vi "MockbusTest.vi"() -> ()   [LabVIEW 2016]
uses:
  Common_RT_ILC/DataTypes/ILCTelemetry.ctl
  Common_RT_ILC/DataTypes/ILCScanRates.ctl
  Common_RT_HPILC/DataTypes/HPTelemetry.ctl
  Common_RT_Modbus/DataTypes/RxFrame.ctl
  Common_RT_HealthAndStatus/RTHealthAndStatus/RTHealthAndStatus.lvclass
  MyHealthAndStatusReadFIFO/MyHealthAndStatusReadFIFO.lvclass
  D:/Code/Common_RT_FPGA/IReadU32FIFO/IReadU32FIFO.lvclass
  MyHealthAndStatusWriteFIFO/MyHealthAndStatusWriteFIFO.lvclass
  D:/Code/Common_RT_FPGA/IWriteU64FIFO/IWriteU64FIFO.lvclass
  ModbusFactory/ModbusFactory.lvclass
  D:/Code/Common_RT_Modbus/IModbusFactory/IModbusFactory.lvclass
  SubnetFactory/SubnetFactory.lvclass
  Subnet/DataTypes/SubnetSettings.ctl
  Common_RT_HPILC/DataTypes/HPSettings.ctl
  Common_RT_ILC/DataTypes/ILCSettings.ctl
  Common_RT_Modbus/IModbusFactory/IModbusFactory.lvclass
  Common_RT_MTILC/DataTypes/MTSettings.ctl
  Common_RT_MDILC/DataTypes/MDSettings.ctl
  Common_RT_MIILC/DataTypes/MISettings.ctl
  ModbusFactory/ModbusFactory.lvclass/ModbusFactory.ctl
  MyHealthAndStatusWriteFIFO/MyHealthAndStatusWriteFIFO.lvclass/MyHealthAndStatusWriteFIFO.ctl
  MyHealthAndStatusReadFIFO/MyHealthAndStatusReadFIFO.lvclass/MyHealthAndStatusReadFIFO.ctl
  Common_RT_HealthAndStatus/RTHealthAndStatus/RTHealthAndStatus.lvclass/RTHealthAndStatus.ctl
  Subnet/Subnet.lvclass/Subnet.ctl
  Common_RT_ILC/ILC/ILC.lvclass/ILC.ctl
  Common_RT_Modbus/DynamicFrameParser/DynamicFrameParser.lvclass
  Common_RT_HPILC/HPILC/HPILC.lvclass/HPILC.ctl
  Common_RT_HPILC/HPILC/HPILC.lvclass
  D:/Code/Common_RT_ILC/ILC/ILC.lvclass
  <vilib>/FPGAPlugInAG/cRIO-9038/niLvFpga_Open_cRIO-9038.vi
  <vilib>/rvi/interface/common/dynamic/niFpgaDynamicAddResources.vi
  <vilib>/FPGAPlugInAG/Dynamic/niLvFpga_Abort_Dynamic.vi
  <vilib>/FPGAPlugInAG/Dynamic/niLvFpga_Reset_Dynamic.vi
  <vilib>/FPGAPlugInAG/Dynamic/niLvFpga_Run_Dynamic.vi
  <vilib>/Utility/error.llb/Error Cluster From Error Code.vi
  <vilib>/rvi/errors/niLvFpgaAdjustHostInterfaceError.vi
  <vilib>/FPGAPlugInAG/Dynamic/niLvFpga_Close_Dynamic.vi
  <vilib>/rvi/interface/nirviOpenFPGA/nirviOpenFPGA.xnode
  FPGA Bitfiles/mockbusTesting.lvbitx
  FPGA/mockbusTesting.vi
  <vilib>/rvi/interface/nirviMethod/nirviMethod.xnode
  <vilib>/rvi/interface/nirviCloseFPGA/nirviCloseFPGA.xnode
  Subnet/Subnet.lvclass
  Common_RT_Modbus/IModbus/IModbus.lvclass
  Common_RT_ILC/RTILC.lvlib
  Common_RT_HPILC/RTHPILC.lvlib
  <vilib>/rvi/errors/niLvFpgaMergeErrorWithErrorCode.vi
  <vilib>/FPGAPlugInAG/Dynamic/niLvFpga_ReadFifo_Dynamic.vi
  Common_RT_MIILC/RTMIILC.lvlib
  Common_RT_MDILC/RTMDILC.lvlib
  Common_RT_MTILC/RTMTILC.lvlib
  <vilib>/FPGAPlugInAG/Dynamic/niLvFpga_WriteFifo_Dynamic.vi
  Common_RT_ILC/ILC/ILC.lvclass
  Common_RT_Modbus/RTModbus.lvlib
panel:
  out "CRCIssues":T1[](array[typedef]) {"Data" format="%02x"}
  in  "BroadcastCounter":u8
  in  "Command.Steps":i8
  out "Telemetry":T2
  out "InvalidCRC":i32
  out "ValidCRC":i32
  out "Array":T3[](array[typedef]) {"ADCScanRate" items=["50 Hz"=0, "60 Hz"=1, "100 Hz"=2, "120 Hz"=3, "200 Hz"=4, "240 Hz"=5, "300 Hz"=6, "400 Hz"=7, "480 Hz"=8, "600 Hz"=9, "1200 Hz"=10, "2400 Hz"=11, "4800 Hz"=12, "No Change"=255]}
  out "Port 2 Status Bits":u64 format="%016b"
  out "Port 2 Frames Received":i64
  out "Port 2 Bytes Received":i64
  out "Port 2 Frames Transmitted":i64
  out "Port 2 Bytes Transmitted":i64
  in  "Boolean":bool
  out "Port 1 Status Bits":u64 format="%016b"
  out "error out":errorcluster
  out "Port 1 Frames Received":i64
  out "Port 1 Bytes Received":i64
  out "Port 1 Frames Transmitted":i64
  out "Port 1 Bytes Transmitted":i64
  # "Port 1 = Modbus"
  # "Port 2 = Mockbus"
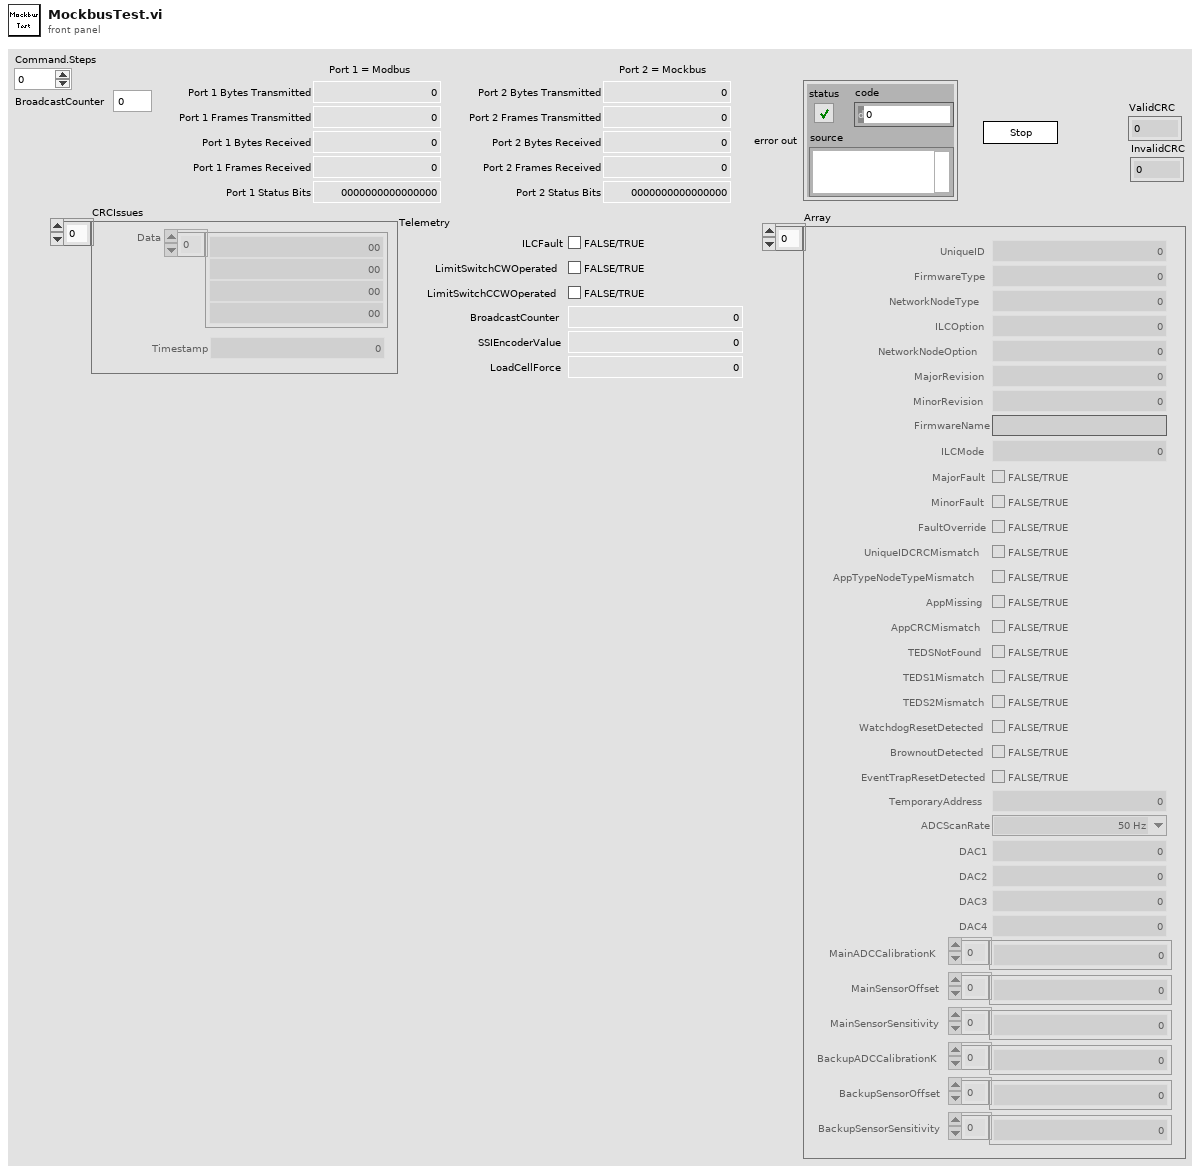
[diagram p1: front panel]
types:
  T1 = typedef "RTModbus.lvlib/RxFrame.ctl" = cluster{"Data":u8[], "Timestamp":u64}
  T2 = typedef "RTHPILC.lvlib/HPTelemetry.ctl" = cluster{"ILCFault":bool, "LimitSwitchCWOperated":bool, "LimitSwitchCCWOperated":bool, "BroadcastCounter":u8, "SSIEncoderValue":i32, "LoadCellForce":sgl}
  T3 = typedef "RTILC.lvlib/ILCTelemetry.ctl" = cluster{"UniqueID":u64, "FirmwareType":u8, "NetworkNodeType":u8, "ILCOption":u8, "NetworkNodeOption":u8, "MajorRevision":u8, "MinorRevision":u8, "FirmwareName":string, "ILCMode":u16, "MajorFault":bool, "MinorFault":bool, "FaultOverride":bool, "UniqueIDCRCMismatch":bool, "AppTypeNodeTypeMismatch":bool, "AppMissing":bool, "AppCRCMismatch":bool, "TEDSNotFound":bool, "TEDS1Mismatch":bool, "TEDS2Mismatch":bool, "WatchdogResetDetected":bool, "BrownoutDetected":bool, "EventTrapResetDetected":bool, "TemporaryAddress":u8, "ADCScanRate":T4, "DAC1":u16, "DAC2":u16, "DAC3":u16, "DAC4":u16, "MainADCCalibrationK":sgl[], "MainSensorOffset":sgl[], "MainSensorSensitivity":sgl[], "BackupADCCalibrationK":sgl[], "BackupSensorOffset":sgl[], "BackupSensorSensitivity":sgl[]}
  T4 = typedef "RTILC.lvlib/ILCScanRates.ctl" = u8
  T5 = typedef "RTHPILC.lvlib/HPSettings.ctl" = cluster{"ILCSettings":T6, "ID":i16, "ReferencePosition":i32}
  T6 = typedef "RTILC.lvlib/ILCSettings.ctl" = cluster{"Subnet":u8, "Address":u8}
  T7 = typedef "SubnetSettings.ctl" = cluster{"HPs":T5[], "ModbusFactory":refnum<class "IModbusFactory.lvclass">, "Port":i32, "MTs":T8[], "MDs":T9[], "MIs":T10[]}
  T8 = typedef "RTMTILC.lvlib/MTSettings.ctl" = cluster{"ILCSettings":T6, "ID":i16}
  T9 = typedef "RTMDILC.lvlib/MDSettings.ctl" = cluster{"ILCSettings":T6, "ID":i16}
  T10 = typedef "RTMIILC.lvlib/MISettings.ctl" = cluster{"ILCSettings":T6, "ID":i16}
  T11 = typedef "SubnetData.ctl" = cluster{"SubnetConstants":T12, "SubnetCommand":T15, "SubnetTelemetry":T16}
  T12 = typedef "SubnetConstants.ctl" = cluster{"Modbus":refnum<class "IModbus.lvclass">, "HPs":refnum<class "HPILC.lvclass">[], "AddressToActuator":T13[], "MTs":refnum<class "MTILC.lvclass">[], "MDs":refnum<class "MDILC.lvclass">[], "MIs":refnum<class "MIILC.lvclass">[]}
  T13 = typedef "ILCIndexData.ctl" = cluster{"ILCTypes":T14, "Index":i32}
  T14 = typedef "ILCTypes.ctl" = enum16{"Undefined", "SAA", "DAA", "HP", "MT", "MD", "MI"}
  T15 = typedef "SubnetCommand.ctl" = cluster{"BroadcastCounter":u8}
  T16 = typedef "SubnetTelemetry.ctl" = cluster{"BytesTransmitted":u32, "FramesTransmitted":u32, "BytesReceived":u32, "FramesReceived":u32, "TxInternalFIFOOverflow":bool, "InvalidInstruction":bool, "WaitForRxFrameTimeout":bool, "StartBitError":bool, "StopBitError":bool, "RxDataFIFOOverflow":bool}
  T17 = typedef "RTILC.lvlib/ILCData.ctl" = cluster{"Constants":T18, "Command":T19, "Telemetry":T3, "Responses":T20, "Timings":T22}
  T18 = typedef "RTILC.lvlib/ILCConstants.ctl" = cluster{"Subnet":u8, "Address":u8}
  T19 = typedef "RTILC.lvlib/ILCCommand.ctl" = cluster{"ILCMode":u16, "TemporaryAddress":u8, "ADCScanRate":T4, "ADCChannel":u8, "ADCOffset":sgl, "ADCSensitivity":sgl}
  T20 = typedef "RTILC.lvlib/ILCResponses.ctl" = cluster{"ReportServerID":T21, "ReportServerStatus":T21, "ILCMode":T21, "SetTemporaryAddress":T21, "Reset":T21, "ADCScanRate":T21, "ADCOffsetSensitivity":T21, "ReadDAC":T21, "ReadCalibration":T21}
  T21 = typedef "RTModbus.lvlib/ExceptionCodes.ctl" = u16
  T22 = typedef "RTILC.lvlib/ILCTimings.ctl" = cluster{"ADCOffsetSensitivity":u32, "ADCScanRate":u32, "ILCMode":u32, "ReadCalibration":u32, "ReportServerID":u32, "ReportServerStatus":u32, "Reset":u32, "SetTemporaryAddress":u32}
  T23 = typedef "RTHPILC.lvlib/HPData.ctl" = cluster{"Constants":T24, "Command":T25, "Telemetry":T2, "Responses":T26, "Timings":T27}
  T24 = typedef "RTHPILC.lvlib/HPConstants.ctl" = cluster{"ID":i16, "ReferencePosition":i32}
  T25 = typedef "RTHPILC.lvlib/HPCommand.ctl" = cluster{"Steps":i8}
  T26 = typedef "RTHPILC.lvlib/HPResponses.ctl" = cluster{"StepMotor":T21, "ForceAndStatus":T21}
  T27 = typedef "RTHPILC.lvlib/HPTimings.ctl" = cluster{"BroadcastStepMotor":u32, "ForceAndStatus":u32, "FreezeSensorValues":u32, "StepMotor":u32}
  T28 = typedef "RTModbus.lvlib/TxFrame.ctl" = cluster{"Data":u8[], "WaitForTrigger":bool, "WaitForRx":u16, "TriggerIRQ":bool, "DelayMicroseconds":u16, "DelayMilliseconds":u16, "Timestamp":bool}
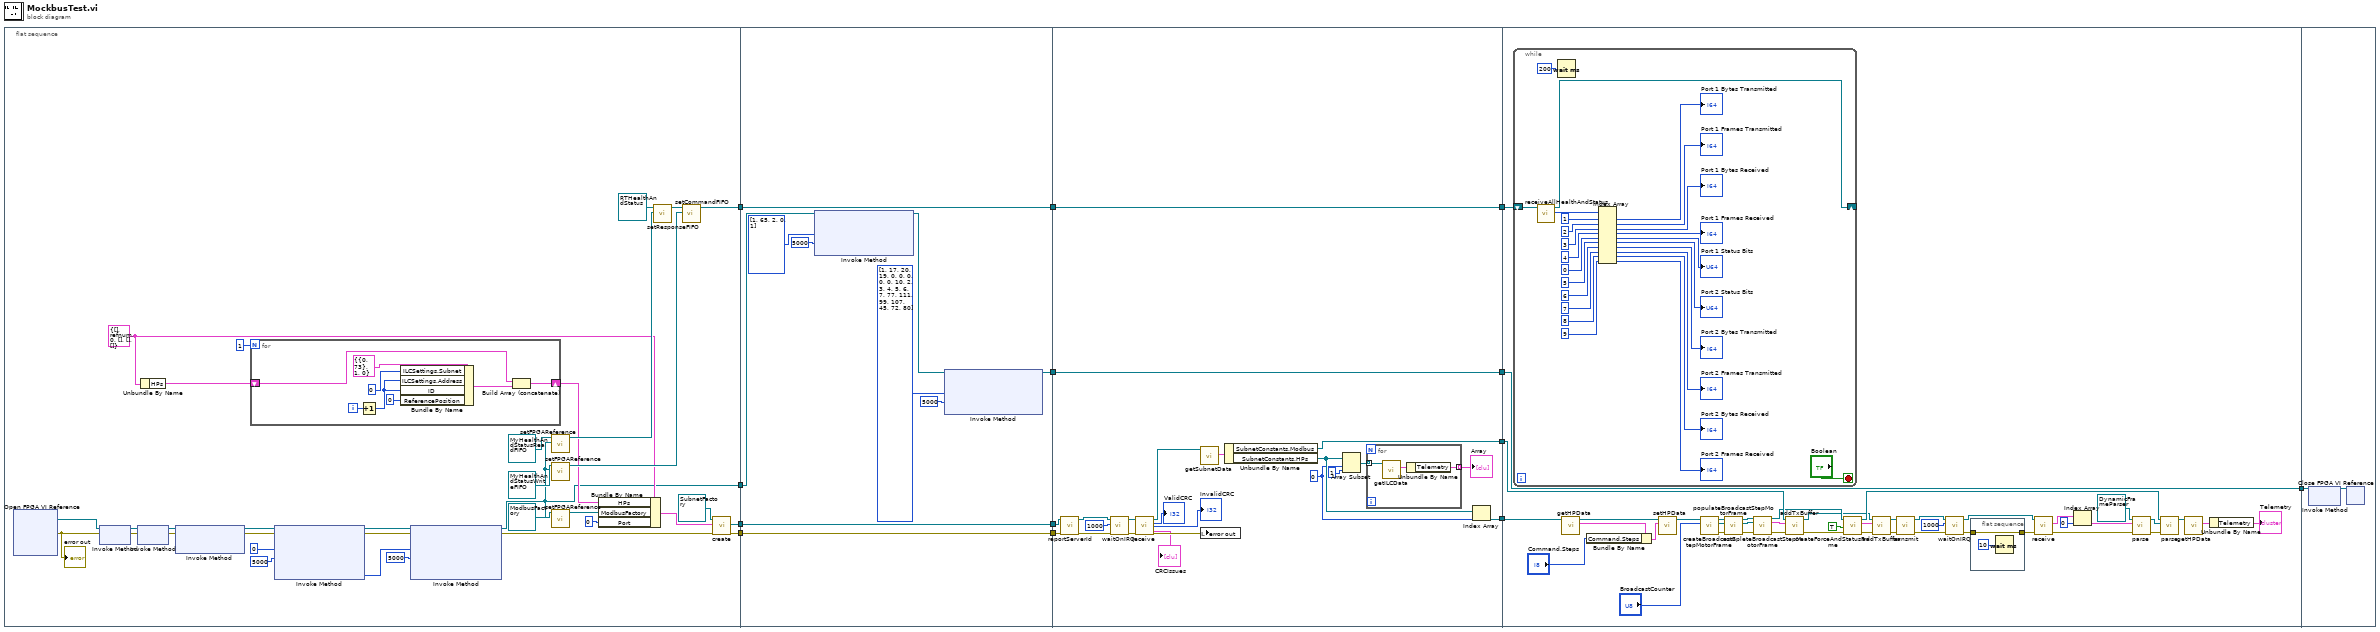
[diagram p0: block diagram]
diagram:
  n1 = flat-sequence {
    tunnel: [w14] -> w12
    tunnel: [w44] -> w10
    tunnel: [w31] -> w8
    tunnel: [w16] -> w6
    tunnel: w12 -> [w62]
    tunnel: [w59] -> w11
    tunnel: w10 -> [w65]
    tunnel: [w65] -> w9
    tunnel: w8 -> [w64]
    tunnel: [w64] -> w7
    tunnel: w6 -> [w63]
    tunnel: [w63] -> w5
    tunnel: w11 -> [w87]
    tunnel: [w87] -> w4
    tunnel: w9 -> [w86]
    tunnel: [w86] -> w3
    tunnel: w7 -> [w72]
    tunnel: w5 -> [w71]
    tunnel: [w68] -> w2
    tunnel: [w67] -> w1
    tunnel: [w132] -> w13
    tunnel: w3 -> [w133]
    tunnel: w4 -> [w132]
    tunnel: w2 -> [w131]
    tunnel: w1 -> [w127]
    tunnel: w13 -> [w161]
    frame #0 {
      w36 = T7 {"HPs"=[], "ModbusFactory"=refnum, "Port"=0, "MTs"=[], "MDs"=[], "MIs"=[]} ("SubnetSettings")
      n2 = xnode "Open FPGA VI Reference"() -> ("FPGA VI Reference Out"=w38:refnum<k20>, "error out"=w18:errorcluster)  [unwired: 2 in]
      "error out" <- w18
      n3 = xnode "Invoke Method"("FPGA VI Reference In"=w38, "error in"=w18) -> ("FPGA VI Reference Out"=w47:refnum<k20>, "error out"=w39:errorcluster)
      n4 = xnode "Invoke Method"("FPGA VI Reference In"=w47, "error in"=w39) -> ("FPGA VI Reference Out"=w24:refnum<k20>, "error out"=w22:errorcluster)
      n5 = Unbundle By Name(w36) -> ("HPs"=w20:T5[])
      n6 = xnode "Invoke Method"("FPGA VI Reference In"=w24, "error in"=w22) -> ("FPGA VI Reference Out"=w23:refnum<k20>, "error out"=w21:errorcluster)  [unwired: 1 in]
      n7 = for {
        N: 1 -> [_]
        shift-right: [w49] -> w19
        shift-left: w20 -> [w50]
        i -> [w54]
        n8 = Increment(x=w54) -> (x+1=w48:i32)
        n9 = Bundle By Name(cluster=T5 {"ILCSettings"={"Subnet"=0, "Address"=73}, "ID"=1, "ReferencePosition"=0} ("HPSettings"), "ILCSettings.Subnet"=u8 0, "ILCSettings.Address"=w48, "ID"=w48, "ReferencePosition"=0) -> (w51:T5)
        n10 = Build Array (concatenate)(w50, w51) -> (w49:T5[])
      }
      n11 = xnode "Invoke Method"("FPGA VI Reference In"=w23, "error in"=w21, "Number of Elements"=u32 0, "Timeout (ms)"=5000) -> ("FPGA VI Reference Out"=w27:refnum<k20>, "error out"=w25:errorcluster, "Elements Remaining"=w28:u32)  [unwired: 1 out]
      n12 = xnode "Invoke Method"("FPGA VI Reference In"=w27, "error in"=w25, "Number of Elements"=w28, "Timeout (ms)"=5000) -> ("FPGA VI Reference Out"=w14:refnum<k20>, "error out"=w17:errorcluster)  [unwired: 2 out]
      n13 = call "setFPGAReference.vi"("FPGAReference"=w14, "MyHealthAndStatusReadFIFO in"=refnum<class "MyHealthAndStatusReadFIFO.lvclass"> refnum ("MyHealthAndStatusReadFIFO.lvclass")) -> ("MyHealthAndStatusReadFIFO out"=w42:refnum<class "MyHealthAndStatusReadFIFO.lvclass">)  [unwired: 9 in]
      n14 = call "setFPGAReference.vi"("FPGAReference"=w14, "MyHealthAndStatusWriteFIFO in"=refnum<class "MyHealthAndStatusWriteFIFO.lvclass"> refnum ("MyHealthAndStatusWriteFIFO.lvclass")) -> ("MyHealthAndStatusWriteFIFO out"=w40:refnum<class "MyHealthAndStatusWriteFIFO.lvclass">)  [unwired: 9 in]
      n15 = call "setFPGAReference.vi"("FPGAReference"=w14, "ModbusFactory in"=refnum<class "ModbusFactory.lvclass"> refnum ("ModbusFactory.lvclass")) -> ("ModbusFactory out"=w34:refnum<class "ModbusFactory.lvclass">)  [unwired: 9 in]
      n16 = Bundle By Name(cluster=w36, "HPs"=w19, "ModbusFactory"=w34, "Port"=0) -> (w33:T7)
      n17 = call "setResponseFIFO.vi"("ReadU32FIFO"=w42, "RTHealthAndStatus in"=refnum<class "RTHealthAndStatus.lvclass"> refnum ("RTHealthAndStatus.lvlib:RTHealthAndStatus.lvclass")) -> ("RTHealthAndStatus out"=w45:refnum<class "RTHealthAndStatus.lvclass">)  [unwired: 9 in]
      n18 = call "setCommandFIFO.vi"("WriteU64FIFO"=w40, "RTHealthAndStatus in"=w45) -> ("RTHealthAndStatus out"=w44:refnum<class "RTHealthAndStatus.lvclass">)  [unwired: 9 in]
      n19 = call "create.vi"("error in (no error)"=w17, "SubnetSettings"=w33, "SubnetFactory in"=refnum<class "SubnetFactory.lvclass"> refnum ("SubnetFactory.lvclass")) -> ("error out"=w16:errorcluster, "Subnet"=w31:refnum<class "Subnet.lvclass">)  [unwired: 6 in, 1 out]
    }
    frame #1 {
      n20 = xnode "Invoke Method"("FPGA VI Reference In"=w62, "Data"=u8[] [1, 65, 2, 0, 1], "Timeout (ms)"=5000) -> ("FPGA VI Reference Out"=w58:refnum<k20>)  [unwired: 1 in, 2 out]
      n21 = xnode "Invoke Method"("FPGA VI Reference In"=w58, "Data"=u8[] [1, 17, 20, 19, 0, 0, 0, 0, 0, 10, 2, 3, 4, 5, 6, 7, 77, 111, 99, 107, 45, 72, 80], "Timeout (ms)"=5000) -> ("FPGA VI Reference Out"=w59:refnum<k20>)  [unwired: 1 in, 2 out]
    }
    frame #2 {
      w69 = 0 ("index")
      n22 = call-dynamic "reportServerId.vi"("error in (no error)"=w71, "Subnet in"=w72) -> ("error out"=w80:errorcluster, "Subnet out"=w81:refnum<class "Subnet.lvclass">)  [unwired: 8 in]
      n23 = call-dynamic "waitOnIRQ.vi"("error in (no error)"=w80, "Timeout (ms)"=1000, "Subnet in"=w81) -> ("error out"=w77:errorcluster, "Subnet out"=w78:refnum<class "Subnet.lvclass">)  [unwired: 7 in]
      n24 = call-dynamic "receive.vi"("Subnet in"=w78, "error in (no error)"=w77) -> ("Subnet out"=w76:refnum<class "Subnet.lvclass">, "ValidCRC"=→"ValidCRC":i32, "InvalidCRC"=→"InvalidCRC":i32, "CRCIssues"=→"CRCIssues":T1[], "error out"=w73:errorcluster)  [unwired: 8 in, 1 out]
      n25 = call "getSubnetData.vi"("Subnet in"=w76) -> ("SubnetData"=w85:T11)  [unwired: 9 in, 1 out]
      n26 = local write "error out"(w73) -> ()
      n27 = Unbundle By Name(w85) -> ("SubnetConstants.Modbus"=w67:refnum<class "IModbus.lvclass">, "SubnetConstants.HPs"=w70:refnum<class "HPILC.lvclass">[])
      n28 = Array Subset(array=w70, index=w69, length=1) -> (w83:refnum<class "HPILC.lvclass">[])
      n29 = for {
        tunnel: w83 -> [w90] mode=indexing
        tunnel: [w88] -> w82 mode=indexing
        n30 = call "getILCData.vi"("ILC in"=w90) -> ("ILCData"=w89:T17)  [unwired: 9 in, 1 out]
        n31 = Unbundle By Name(w89) -> ("Telemetry"=w88:T3)
      }
      "Array" <- w82
      n32 = Index Array(array=w70, index=w69) -> (element=w68:refnum<class "HPILC.lvclass">)
    }
    frame #3 {
      n33 = while {
        shift-right: [w158] -> _
        shift-left: w133 -> [w159]
        stop <- "Boolean" stop-if-true
        n34 = call "receiveAllHealthAndStatus.vi"("RTHealthAndStatus in"=w159) -> ("Data"=w153:u32[], "RTHealthAndStatus out"=w158:refnum<class "RTHealthAndStatus.lvclass">)  [unwired: 8 in, 1 out]
        n35 = Wait (ms)(milliseconds to wait=u32 200) -> ()  [unwired: 1 out]
        n36 = Index Array(array=w153, index #1=1 ("index"), index #2=2 ("index"), index #3=3 ("index"), index #4=4 ("index"), index #5=0 ("index"), index #6=5 ("index"), index #7=6 ("index"), index #8=7 ("index"), index #9=8 ("index"), index #10=9 ("index")) -> (element #1=→"Port 1 Bytes Transmitted":u32, element #2=→"Port 1 Frames Transmitted":u32, element #3=→"Port 1 Bytes Received":u32, element #4=→"Port 1 Frames Received":u32, element #5=→"Port 1 Status Bits":u32, element #6=→"Port 2 Status Bits":u32, element #7=→"Port 2 Bytes Transmitted":u32, element #8=→"Port 2 Frames Transmitted":u32, element #9=→"Port 2 Bytes Received":u32, element #10=→"Port 2 Frames Received":u32)
      }
      n37 = call "getHPData.vi"("HPILC in"=w131) -> ("HPData"=w130:T23, "HPILC out"=w128:refnum<class "HPILC.lvclass">)  [unwired: 9 in]
      n38 = Bundle By Name(cluster=w130, "Command.Steps"="Command.Steps") -> (w129:T23)
      n39 = call "setHPData.vi"("HPData"=w129, "HPILC in"=w128) -> ("HPILC out"=w109:refnum<class "HPILC.lvclass">)  [unwired: 9 in]
      n40 = call "createBroadcastStepMotorFrame.vi"("BroadcastCounter"="BroadcastCounter", "HPILC in"=w109) -> ("error out"=w100:errorcluster, "FixedFrameBuilder"=w106:refnum<class "FixedFrameBuilder.lvclass">, "HPILC out"=w107:refnum<class "HPILC.lvclass">)  [unwired: 7 in]
      n41 = call "populateBroadcastStepMotorFrame.vi"("error in (no error)"=w100, "FixedFrameBuilder in"=w106, "HPILC in"=w107) -> ("error out"=w101:errorcluster, "FixedFrameBuilder out"=w104:refnum<class "FixedFrameBuilder.lvclass">, "HPILC out"=w105:refnum<class "HPILC.lvclass">)  [unwired: 6 in]
      n42 = call "completeBroadcastStepMotorFrame.vi"("HPILC in"=w105, "FixedFrameBuilder"=w104, "error in (no error)"=w101) -> ("HPILC out"=w98:refnum<class "HPILC.lvclass">, "TxFrame"=w103:T28, "error out"=w102:errorcluster)  [unwired: 10 in]
      n43 = call-dynamic "addTxBuffer.vi"("error in (no error)"=w102, "TxFrame"=w103, "IModbus in"=w127) -> ("error out"=w97:errorcluster, "IModbus out"=w92:refnum<class "IModbus.lvclass">)  [unwired: 7 in]
      n44 = call "createForceAndStatusFrame.vi"("error in (no error)"=w97, "TriggerIRQ"=TRUE, "HPILC in"=w98) -> ("error out"=w96:errorcluster, "TxFrame"=w95:T28, "HPILC out"=w94:refnum<class "HPILC.lvclass">)  [unwired: 6 in]
      n45 = call-dynamic "addTxBuffer.vi"("error in (no error)"=w96, "TxFrame"=w95, "IModbus in"=w92) -> ("error out"=w91:errorcluster, "IModbus out"=w93:refnum<class "IModbus.lvclass">)  [unwired: 7 in]
      n46 = call-dynamic "transmit.vi"("error in (no error)"=w91, "IModbus in"=w93) -> ("error out"=w124:errorcluster, "IModbus out"=w126:refnum<class "IModbus.lvclass">)  [unwired: 8 in]
      n47 = call-dynamic "waitOnIRQ.vi"("error in (no error)"=w124, "Timeout"=1000, "IModbus in"=w126) -> ("error out"=w111:errorcluster, "IModbus out"=w123:refnum<class "IModbus.lvclass">)  [unwired: 5 in, 2 out]
      n48 = flat-sequence {
        tunnel: [w134] -> w112
        tunnel: w111 -> [w134]
        frame #0 {
          n49 = Wait (ms)(milliseconds to wait=u32 10) -> ()  [unwired: 1 out]
        }
      }
      n50 = call-dynamic "receive.vi"("error in (no error)"=w112, "IModbus in"=w123) -> ("error out"=w113:errorcluster, "Data"=w122:T1[])  [unwired: 7 in, 1 out]
      n51 = Index Array(array=w122, index=0) -> (element=w120:T1)
      n52 = call "parse.vi"("error in (no error)"=w113, "RxFrame"=w120, "FrameParser in"=refnum<class "DynamicFrameParser.lvclass"> refnum ("RTModbus.lvlib:DynamicFrameParser.lvclass")) -> ("error out"=w114:errorcluster, "FrameParser out"=w118:refnum<class "DynamicFrameParser.lvclass">)  [unwired: 7 in]
      n53 = call-dynamic "parse.vi"("error in (no error)"=w114, "DynamicFrameParser"=w118, "HPILC in"=w94) -> ("HPILC out"=w117:refnum<class "HPILC.lvclass">)  [unwired: 6 in, 2 out]
      n54 = call "getHPData.vi"("HPILC in"=w117) -> ("HPData"=w116:T23)  [unwired: 9 in, 1 out]
      n55 = Unbundle By Name(w116) -> ("Telemetry"=→"Telemetry":T2)
    }
    frame #4 {
      n56 = xnode "Invoke Method"("FPGA VI Reference In"=w161) -> ("FPGA VI Reference Out"=w162:refnum<k20>)  [unwired: 1 in, 1 out]
      n57 = xnode "Close FPGA VI Reference"("FPGA VI Reference In"=w162) -> ()  [unwired: 1 in, 1 out]
    }
  }
